vi "Read Topic Info.vi"(11 "Topic in":refnum<class "Topic.lvclass">) -> (0 "Last Publication Time":timestamp, 1 "Enqueuer (UID)":refnum<class "Message Enqueuer.lvclass">, 2 "Name":string, 3 "Type":string)   [LabVIEW 2018, in "MVA Framework.lvlib" / "Mediator.lvlib" / "Topic.lvclass"]
doc: "读取主题信息"
uses:
  Topic.lvclass
  <vilib>/ActorFramework/Actor/Actor.lvclass
  <vilib>/ActorFramework/Message Enqueuer/Message Enqueuer.lvclass
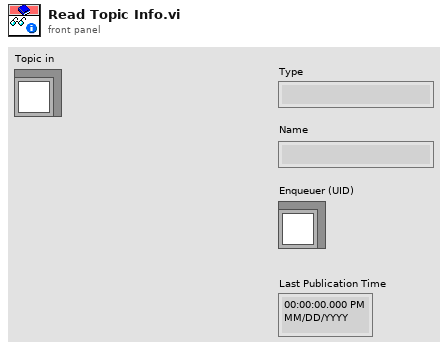
[diagram p1: front panel]
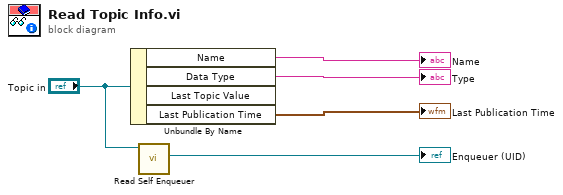
[diagram p0: block diagram]
diagram:
  n1 = Unbundle By Name("Topic in") -> ("Name"=→"Name":string, "Data Type"=→"Type":string, "Last Publication Time"=→"Last Publication Time":timestamp)  [unwired: 1 out]
  n2 = call <vilib>:"Read Self Enqueuer.vi"("Actor"="Topic in") -> ("Self Enqueuer"=→"Enqueuer (UID)":refnum<class "Message Enqueuer.lvclass">)  [unwired: 10 in]
